vi "Global GPS.vi"() -> ()   [LabVIEW 2015]
panel:
  out "GPS Data":T1
  in  "output cluster":T2
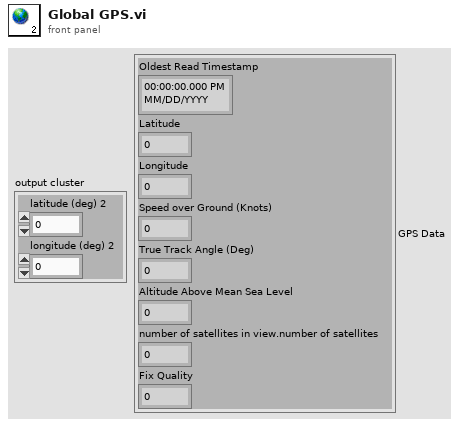
[diagram p1: front panel]
types:
  T1 = cluster{"Oldest Read Timestamp":timestamp, "Latitude":dbl, "Longitude":dbl, "Speed over Ground (Knots)":dbl, "True Track Angle (Deg)":dbl, "Altitude Above Mean Sea Level":dbl, "number of satellites in view.number of satellites":i8, "Fix Quality ":u16}
  T2 = cluster{"latitude (deg) 2":dbl, "longitude (deg) 2":dbl}
diagram:
